vi "Teleop.vi"(10 "Match Info":T1={"Autonomous Elapsed Seconds"=0.0, "TeleOp Elapsed Seconds"=0.0, "Disabled Elapsed Seconds"=0.0, "Visited Autonomous"=FALSE, "Visited TeleOp"=FALSE, "Visited Disabled"=FALSE, "Autonomous Settings"={"Autonomous Style"=enum."Independent", "VI Refnum"=refnum}}, 11 "Call Context":T2) -> ()   [LabVIEW 2017]
doc: "This VI is called for each enabled TeleOp packet received from the DS. It is typically used to read from joysticks and other inputs and update I/O or setpoints for timed control loops. It should complete and return within 20 milliseconds or risk missing DS packets."
uses:
  <vilib>/Rock Robotics/WPI/DriverStation/WPI_DriverStationDerivedRobotMode.ctl
  <vilib>/Rock Robotics/WPI/DriverStation/WPI_DriverStationMatch Info.ctl
  <vilib>/Rock Robotics/WPI/Utilities/WPI_GetSetVariantRefNum.vi
  <vilib>/Rock Robotics/Network Tables/NT Write Boolean Array.vi
  <vilib>/Rock Robotics/Network Tables/NT Write Numeric Array.vi
panel:
  in  "Drive":enum16{"Cheesy", "Tank"}(ring)
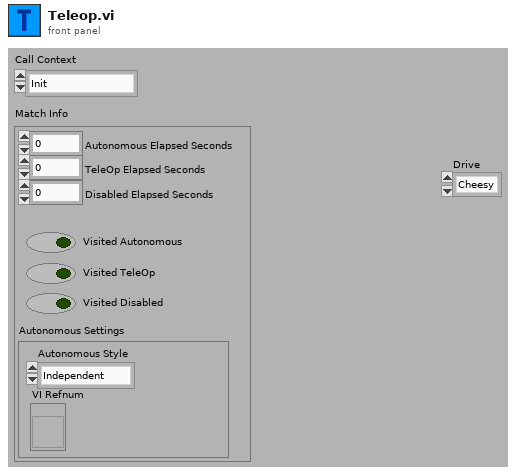
[diagram p1: front panel]
types:
  T1 = typedef "WPI_DriverStationMatch Info.ctl" = cluster{"Autonomous Elapsed Seconds":dbl, "TeleOp Elapsed Seconds":dbl, "Disabled Elapsed Seconds":dbl, "Visited Autonomous":bool, "Visited TeleOp":bool, "Visited Disabled":bool, "Autonomous Settings":cluster{"Autonomous Style":enum16{"Iterative", "Independent"}, "VI Refnum":refnum<vi>}}
  T2 = typedef "WPI_DriverStationDerivedRobotMode.ctl" = enum16{"Init", "Execute", "Stop"}
  T3 = typedef "WPI_JoystickDevRef.ctl" = cluster{"Device":T4}
  T4 = typedef "WPI_JoystickDeviceEnum.ctl" = enum16{"USB 0", "USB 1", "USB 2", "USB 3", "USB 4", "USB 5"}
  T5 = typedef "Command Status Info.ctl" = cluster{"Name":string, "Status":T6, "notifier out":T7}
  T6 = typedef "Completion Status.ctl" = enum16{"Successful", "Aborted", "Incomplete"}
  T7 = typedef "Completion Notifier.ctl" = refnum<notifier>
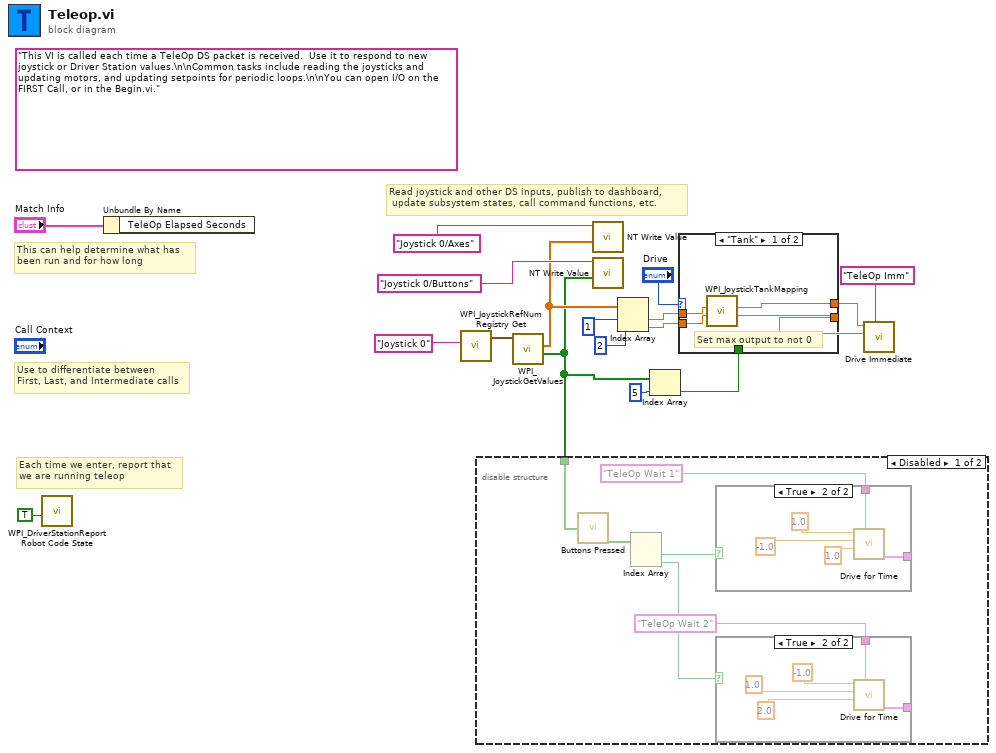
[diagram p0: block diagram]
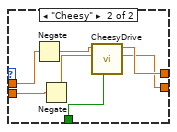
[diagram p2: hidden frame]
diagram:
  (unwired) "This VI is called each time a TeleOp DS packet is received.  Use it to respond to new joystick or Driver Station values.\n\nCommon tasks include reading the joysticks and updating motors, and updating setpoints for periodic loops.\n\nYou can open I/O on the FIRST Call, or in the Begin.vi."
  # "Read joystick and other DS inputs, publish to dashboard,\n update subsystem states, call command functions, etc."
  # "Each time we enter, report that\nwe are running teleop"
  # "Use to differentiate between\nFirst, Last, and Intermediate calls"
  # "This can help determine what has\nbeen run and for how long"
  n1 = call <vilib>:"WPI_DriverStationReport Robot Code State.vi"("TeleOp"=TRUE ("Autonomous")) -> ()  [unwired: 10 in, 1 out]
  n2 = Unbundle By Name("Match Info") -> ()  [unwired: 1 out]
  n3 = call <vilib>:"WPI_JoystickRefNum Registry Get.vi"("refnum name"="Joystick 0") -> ("JoystickDevRef"=w15:T3)  [unwired: 1 in, 9 out]
  n4 = call <vilib>:"WPI_JoystickGetValues.vi"("JoystickDevRef"=w15) -> ("Buttons"=w6:bool[], "Axes"=w12:dbl[])  [unwired: 6 in, 3 out]
  n5 = disable-structure shown="Disabled" {
    disable-tunnel: w6 -> [w20 _]
    frame Disabled {
      n6 = call "Buttons Pressed.vi"("Button Values"=w20) -> ("Button Presses"=w23:bool[])
      n7 = Index Array(array=w23) -> (element #1=w22:bool, element #2=w21:bool)  [unwired: 2 in]
      n8 = case shown="True" w22 {
        tunnel: [_ w28] -> _
        tunnel: "TeleOp Wait 1" ("Description") -> [_ w27]
        frame False {
        }
        frame True {
          n9 = call "Drive for Time.vi"("Description"=w27, "Seconds"=1.0, "Right Speed"=-1.0, "Left Speed"=1.0) -> ("Command Info Out"=w28:T5)  [unwired: 6 in, 1 out]
        }
      }
      n10 = case shown="True" w21 {
        tunnel: [_ w32] -> _
        tunnel: "TeleOp Wait 2" ("Description") -> [_ w31]
        frame False {
        }
        frame True {
          n11 = call "Drive for Time.vi"("Description"=w31, "Seconds"=2.0, "Right Speed"=1.0, "Left Speed"=-1.0) -> ("Command Info Out"=w32:T5)  [unwired: 6 in, 1 out]
        }
      }
    }
    frame Enabled {
    }
  }
  n12 = call-poly <vilib>:"NT Write Value.vi"("Numeric Array"=w12, "Name"="Joystick 0/Axes") -> ()  [unwired: 9 in, 1 out]
  n13 = call-poly <vilib>:"NT Write Value.vi"("Boolean Array"=w6, "Name"="Joystick 0/Buttons") -> ()  [unwired: 9 in, 1 out]
  n14 = Index Array(array=w12, index #1=1 ("index"), index #2=2 ("index")) -> (element #1=w8:dbl, element #2=w7:dbl)
  n15 = Index Array(array=w6, index=5) -> (element=w5:bool)
  n16 = case shown="\"Tank\"" "Drive" {
    tunnel: w8 -> [w38 w42]
    tunnel: w7 -> [w37 w40]
    tunnel: w5 -> [_ w45]
    tunnel: [w36 w44] -> w4
    tunnel: [w35 w43] -> w3
    frame "Tank" {
      # "Set max output to not 0"
      n17 = call <vilib>:"WPI_JoystickTankMapping.vi"("Right axis value"=w37, "Left axis value"=w38) -> ("Right Motor Value"=w35:dbl, "Left Motor Value"=w36:dbl)  [unwired: 8 in]
    }
    frame "Cheesy" {
      n18 = Negate(x=w42) -> (-x=w41:dbl)
      n19 = Negate(x=w40) -> (-x=w39:dbl)
      n20 = call "CheesyDrive.vi"("Quickturn"=w45, "Wheel"=w39, "Throttle"=w41) -> ("Right PWM"=w43:dbl, "Left PWM"=w44:dbl)  [unwired: 7 in]
    }
  }
  n21 = call "Drive Immediate.vi"("Description"="TeleOp Imm", "Right Setpoint"=w3, "Left Setpoint"=w4) -> ()  [unwired: 8 in, 1 out]
